vi "solar_gbl Create Refnums.vi"(4 "Menu":refnum<k9>, 6 "VI":refnum<vi>, 8 "error in (no error)":errorcluster, 10 "Name in":string, 11 "SOLAR in":T1) -> (0 "error out":errorcluster, 1 "Queue":refnum<queue>, 2 "Name out":string, 3 "SOLAR out":T1)   [LabVIEW 2018]
doc: "This creates the target's references including a queue, user event and data value refnum. If the target name is not defined, this sets the name as 'UNKNOWNx' where x is the next target number."
uses:
  solar_ctl Target Global.ctl
  solar_ctl SOLAR Global.ctl
  voyager/solar_voy_ctl Voyager Refnum.ctl
  qtimer/solar_qtimer_ctl Refnum.ctl
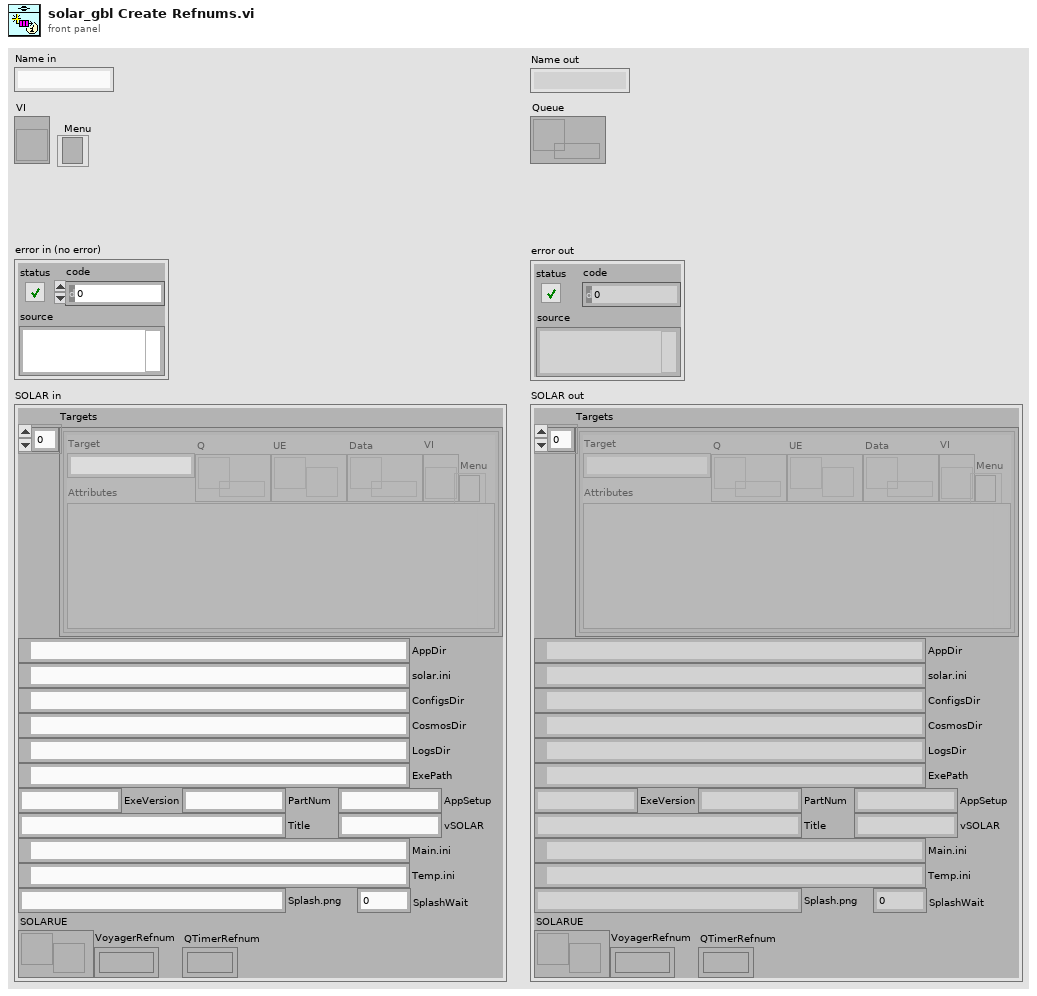
[diagram p1: front panel]
types:
  T1 = typedef "solar_ctl SOLAR Global.ctl" = cluster{"Targets":T2[], "AppDir":path, "solar.ini":path, "ConfigsDir":path, "CosmosDir":path, "LogsDir":path, "ExePath":path, "ExeVersion":string, "PartNum":string, "AppSetup":string, "Title":string, "Main.ini":path, "Temp.ini":path, "vSOLAR":string, "Splash.png":string, "SplashWait":i32, "SOLARUE":refnum<user-event>, "VoyagerRefnum":T3, "QTimerRefnum":T4}
  T2 = typedef "solar_ctl Target Global.ctl" = cluster{"Target":string, "Q":refnum<queue>, "UE":refnum<user-event>, "VI":refnum<vi>, "Menu":refnum<k9>, "Data":refnum<data-value>, "Attributes":variant}
  T3 = typedef "solar_voy_ctl Voyager Refnum.ctl" = refnum<k1>
  T4 = typedef "solar_qtimer_ctl Refnum.ctl" = refnum<k1>
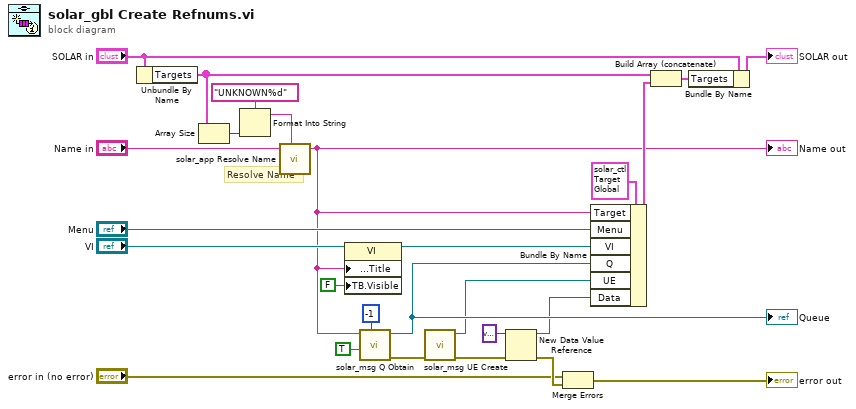
[diagram p0: block diagram]
diagram:
  # "Resolve Name"
  n1 = Unbundle By Name("SOLAR in") -> ("Targets"=w9:T2[])
  n2 = Array Size(array=w9) -> (size(s)=w3:i32)
  n3 = Format Into String(format string="UNKNOWN%d", w3) -> (resulting string=w1:string)  [unwired: 2 in, 1 out]
  n4 = call "solar_app Resolve Name.vi"("Name to Resolve (\"\"=default Name)"="Name in", "default Name"=w1) -> ("Resolved Name"=w4:string)  [unwired: 7 in]
  "Name out" <- w4
  n5 = property class="VI"(reference="VI", "Front Panel.Title"=w4, "TB.Visible"=FALSE ("Tool Bar:Visible")) -> (reference out=w6:refnum<vi>)  [unwired: 1 in, 1 out]
  n6 = call "solar_msg Q Obtain.vi"("Max Queue Size (-1, unlimited)"=-1, "Create If Not Found? (T)"=TRUE, "Queue Name (unnamed)"=w4) -> ("error out"=w18:errorcluster, "Queue"=w21:refnum<queue>)  [unwired: 6 in, 1 out]
  "Queue" <- w21
  n7 = call "solar_msg UE Create.vi"("error in (no error)"=w18) -> ("error out"=w13:errorcluster, "UserEvent"=w17:refnum<user-event>)  [unwired: 9 in]
  n8 = New Data Value Reference(data value=variant ("Data"), error in=w13) -> (data value reference=w14:refnum<data-value>, error out=w12:errorcluster)
  n9 = Merge Errors("error in (no error)", w12) -> (→"error out":errorcluster)
  n10 = Bundle By Name(cluster=T2 {"Target"="", "Q"=refnum, "UE"=refnum, "VI"=refnum, "Menu"=refnum, "Data"=refnum, "Attributes"=variant} ("Target"), "Target"=w4, "Menu"="Menu", "VI"=w6, "Q"=w21, "UE"=w17, "Data"=w14) -> (w22:T2)
  n11 = Build Array (concatenate)(w9, w22) -> (w24:T2[])
  n12 = Bundle By Name(cluster="SOLAR in", "Targets"=w24) -> (→"SOLAR out":T1)
